vi "Unregister Message.vi"(8 "error in (no error)":errorcluster, 10 "View Enqueuer":refnum<class "Message Enqueuer.lvclass">, 11 "Waiting Dialog View in":refnum<class "Waiting Dialog View.lvclass">) -> (0 "error out":errorcluster, 3 "Waiting Dialog View out":refnum<class "Waiting Dialog View.lvclass">)   [LabVIEW 2015, in "Waiting Dialog View.lvlib" / "Waiting Dialog View.lvclass"]
uses:
  Waiting Dialog View.lvclass
  <vilib>/ActorFramework/Message Enqueuer/Message Enqueuer.lvclass
  Waiting Dialog View.lvclass/Waiting Dialog View.ctl
  <vilib>/ActorFrameworkObserver/Actor Register/Actor Register.lvclass
panel:
  # "NOTICE -- YOU MUST LEAVE THIS NOTICE IN PLACE.\n\nCopyright (c) 2015, LIANG LIU Shawn.Liu.cn@gmail.com\nAll rights reserved.\n\nRedistribution and use in source and binary forms, with or without modification, are permitted provided that the following conditions are met:\n-Redistributions of source code must retain the above copyright notice, this list of conditions and the following disclaimer.\n-Redistributions in binary form must reproduce the above copyright notice, this list of conditions and the following disclaimer in the documentation and/or other materials provided with the distribution.\n-Neither the name of the eLp nor the names of its contributors may be used to endorse or promote products derived from this software without specific prior written permission.\n\nTHIS SOFTWARE IS PROVIDED BY THE COPYRIGHT HOLDERS AND CONTRIBUTORS \"AS IS\" AND ANY EXPRESS OR IMPLIED WARRANTIES, INCLUDING, BUT NOT LIMITED TO, THE IMPLIED WARRANTIES OF MERCHANTABILITY AND FITNESS FOR A PARTICULAR PURPOSE ARE DISCLAIMED. IN NO EVENT SHALL THE COPYRIGHT HOLDER OR CONTRIBUTORS BE LIABLE FOR ANY DIRECT, INDIRECT, INCIDENTAL, SPECIAL, EXEMPLARY, OR CONSEQUENTIAL DAMAGES (INCLUDING, BUT NOT LIMITED TO, PROCUREMENT OF SUBSTITUTE GOODS OR SERVICES; LOSS OF USE, DATA, OR PROFITS; OR BUSINESS INTERRUPTION) HOWEVER CAUSED AND ON ANY THEORY OF LIABILITY, WHETHER IN CONTRACT, STRICT LIABILITY, OR TORT (INCLUDING NEGLIGENCE OR OTHERWISE) ARISING IN ANY WAY OUT OF THE USE OF THIS SOFTWARE, EVEN IF ADVISED OF THE POSSIBILITY OF SUCH DAMAGE."
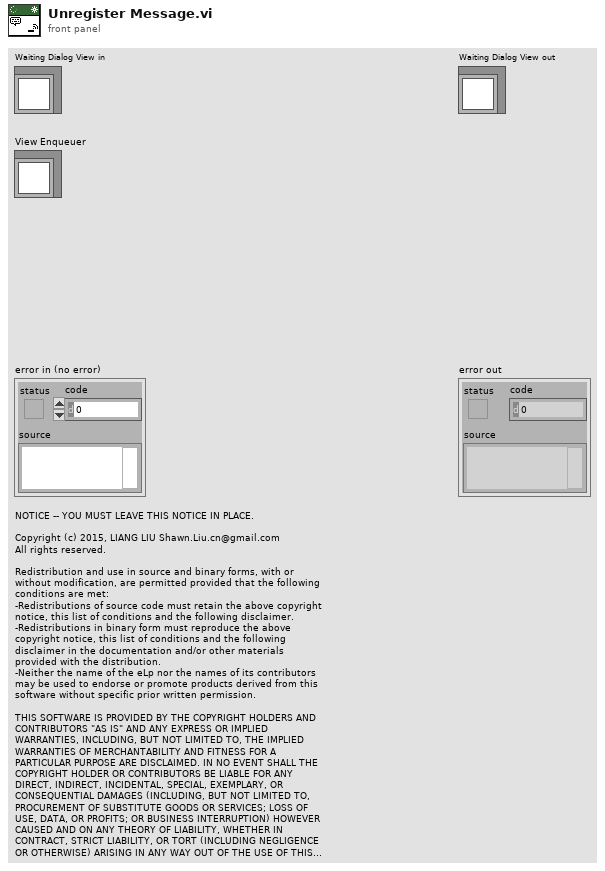
[diagram p1: front panel]
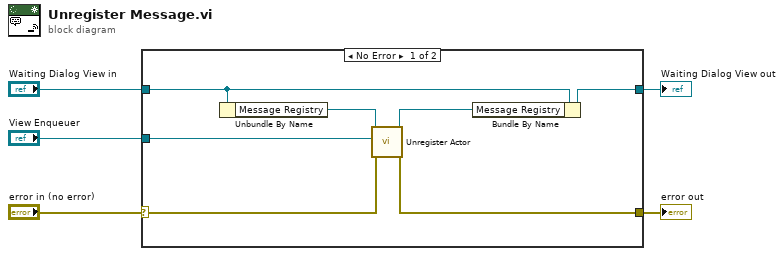
[diagram p0: block diagram]
diagram:
  n1 = case shown="No Error" "error in (no error)" {
    selector: "error in (no error)" -> [w10 w14]
    tunnel: "View Enqueuer" -> [w8 _]
    tunnel: "Waiting Dialog View in" -> [w12 w13]
    tunnel: [w11 w13] -> w1
    tunnel: [w9 w14] -> w3
    frame No Error {
      n2 = Unbundle By Name(w12) -> ("Message Registry"=w7:refnum<class "Actor Register.lvclass">)
      n3 = call <vilib>:"Unregister Actor.vi"("error in (no error)"=w10, "Actor Enqueuer"=w8, "Actor Register in"=w7) -> ("error out"=w9:errorcluster, "Actor Register out"=w6:refnum<class "Actor Register.lvclass">)  [unwired: 7 in]
      n4 = Bundle By Name(cluster=w12, "Message Registry"=w6) -> (w11:refnum<class "Waiting Dialog View.lvclass">)
    }
    frame Error {
    }
  }
  "error out" <- w3
  "Waiting Dialog View out" <- w1
